vi "get sdf root.vi"(8 "error in (no error)":errorcluster, 11 "abstract-tree in":refnum<class "abstract-tree.lvclass">) -> (0 "error out":errorcluster, 1 "sdf root":refnum<k24>, 3 "abstract-tree out":refnum<class "abstract-tree.lvclass">)   [LabVIEW 2017, in "vs-tree-utility.lvlib" / "abstract-tree.lvclass"]
uses:
  abstract-tree.lvclass
  NationalInstruments.VeriStand.SystemDefinitionAPI
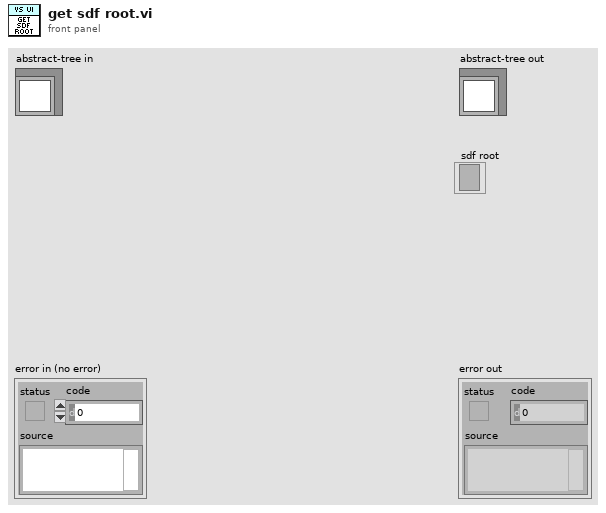
[diagram p1: front panel]
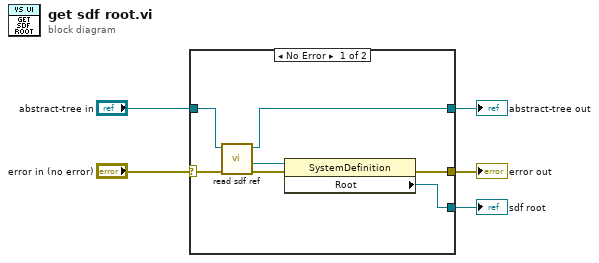
[diagram p0: block diagram]
diagram:
  n1 = case shown="No Error" "error in (no error)" {
    selector: "error in (no error)" -> [w12 w14]
    tunnel: [w10 w14] -> w4
    tunnel: [w6 w13] -> w2
    tunnel: "abstract-tree in" -> [w7 w13]
    tunnel: [w8 _] -> w1
    frame No Error {
      n2 = call-dynamic "read sdf ref.vi"("error in (no error)"=w12, "abstract-tree in"=w7) -> ("error out"=w11:errorcluster, "sdf ref"=w9:refnum<k24>, "abstract-tree out"=w6:refnum<class "abstract-tree.lvclass">)  [unwired: 7 in]
      n3 = property class="SystemDefinition"(reference=w9, error in=w11) -> (error out=w10:errorcluster, "Root"=w8:refnum<k24>)  [unwired: 1 out]
    }
    frame Error {
    }
  }
  "error out" <- w4
  "abstract-tree out" <- w2
  "sdf root" <- w1
